vi "HGF_ThreadPool.appendData2Variant.vi"(0 "initData":variant, 1 "HGF_ThreadWorker":refnum<class "HGF_ThreadWorker.lvclass">, 2 "initialNofThreads (0)":i32, 3 "incThreads(1)":i32=1, 4 "maxNofThreads (-1:unlimited)":i32=-1, 5 "error in (no error)":errorcluster, 7 "autoIncrementLimit (-1)":i32=-1) -> (14 "dup initData":variant, 19 "error out":errorcluster)   [LabVIEW 2014, in "HGF_BaseClasses.lvlib" / "HGF_ThreadPool.lvclass"]
doc: "Append initialize data to variant."
uses:
  HGF_ThreadPool.lvclass
  HGF_ThreadWorker/HGF_ThreadWorker.lvclass
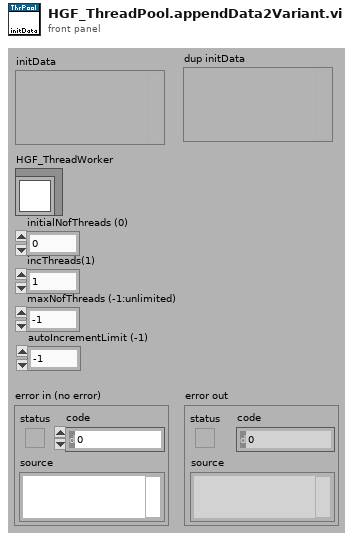
[diagram p1: front panel]
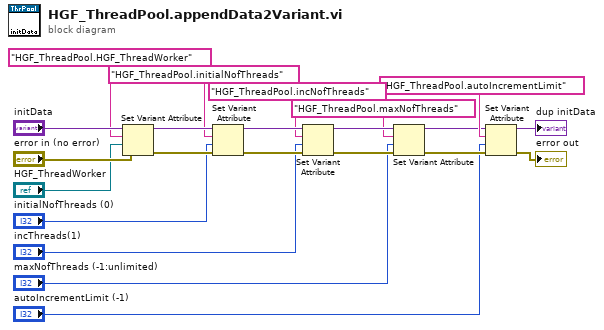
[diagram p0: block diagram]
diagram:
  n1 = Set Variant Attribute(Variant="initData", name="HGF_ThreadPool.HGF_ThreadWorker", value="HGF_ThreadWorker", error in="error in (no error)") -> (Variant out=w18:variant, error out=w16:errorcluster)  [unwired: 1 out]
  n2 = Set Variant Attribute(Variant=w18, name="HGF_ThreadPool.initialNofThreads", value="initialNofThreads (0)", error in=w16) -> (Variant out=w17:variant, error out=w15:errorcluster)  [unwired: 1 out]
  n3 = Set Variant Attribute(Variant=w17, name="HGF_ThreadPool.incNofThreads", value="incThreads(1)", error in=w15) -> (Variant out=w11:variant, error out=w10:errorcluster)  [unwired: 1 out]
  n4 = Set Variant Attribute(Variant=w11, name="HGF_ThreadPool.maxNofThreads", value="maxNofThreads (-1:unlimited)", error in=w10) -> (Variant out=w5:variant, error out=w4:errorcluster)  [unwired: 1 out]
  n5 = Set Variant Attribute(Variant=w5, name="HGF_ThreadPool.autoIncrementLimit", value="autoIncrementLimit (-1)", error in=w4) -> (Variant out=→"dup initData":variant, error out=→"error out":errorcluster)  [unwired: 1 out]
